vi "Queue Dequeue Element.vi"(0 "Queue In":refnum<queue>, 5 "Error In":errorcluster, 16 "State Array":cluster{"State":string}[](array[cluster])) -> (14 "Queue Out":refnum<queue>, 19 "Error Out":errorcluster)   [LabVIEW 2015]
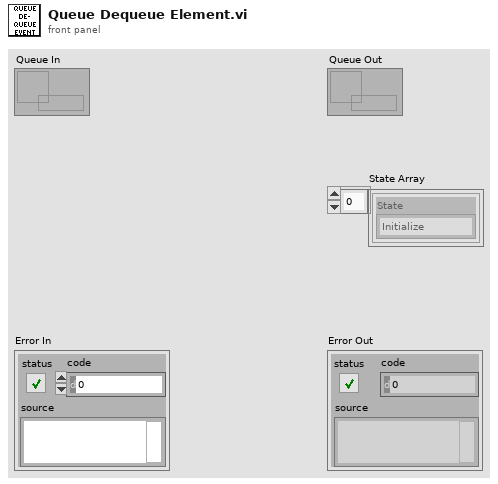
[diagram p1: front panel]
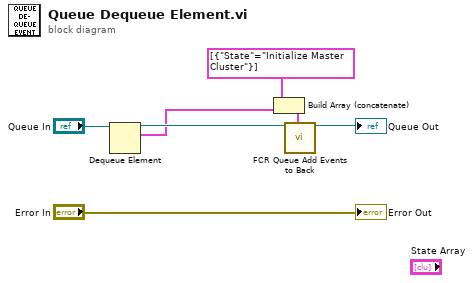
[diagram p0: block diagram]
diagram:
  n1 = Dequeue Element(queue="Queue In") -> (queue out=w5:refnum<queue>, element=w2:cluster{"State":string})  [unwired: 2 in, 2 out]
  n2 = Build Array (concatenate)(cluster{"State":string}[] [{"State"="Initialize Master Cluster"}], w2) -> (w4:cluster{"State":string}[])
  n3 = call "FCR Queue Add Events to Back.vi"("Queue In"=w5, "State Array"=w4) -> ("Queue Out"=→"Queue Out":refnum<queue>)  [unwired: 16 in, 1 out]
  "Error Out" <- "Error In"
